vi "Clean Up.vi"(8 "error in (no error)":errorcluster, 11 "Dell Webcam in":refnum<class "Webcam.lvclass">) -> (0 "error out":errorcluster, 3 "Dell Webcam out":refnum<class "Webcam.lvclass">)   [LabVIEW 2018, in "Webcam.lvclass"]
uses:
  Webcam.lvclass
  Webcam.lvclass/Webcam.ctl
  <vilib>/vision/driver/NI_Vision_Acquisition_Software.lvlib
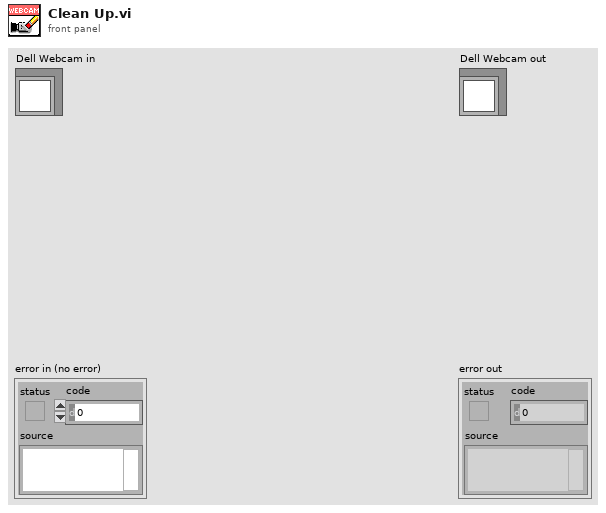
[diagram p1: front panel]
types:
  T1 = typedef "IMAQdx.ctl" = refnum<k21>
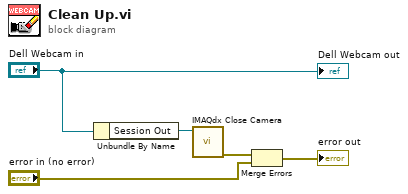
[diagram p0: block diagram]
diagram:
  n1 = Unbundle By Name("Dell Webcam in") -> ("Session Out"=w2:T1)
  n2 = call <vilib>:"IMAQdx Close Camera.vi"("Session In"=w2) -> ("error out"=w5:errorcluster)  [unwired: 1 in, 9 out]
  n3 = Merge Errors(w5, "error in (no error)") -> (→"error out":errorcluster)
  "Dell Webcam out" <- "Dell Webcam in"
